vi "Set Properties.vi"(5 "Group name":string, 7 "Channel name":string, 8 "error in":errorcluster, 9 "Property values":variant[](array[variant]), 10 "Property names":string[](array[string])) -> (0 "error out":errorcluster)   [LabVIEW 2024, in "Data Logger v2.lvlib"]
doc: "Sets the properties of the TDMS file. If group and channel are no values, properties are set at the file level. If channel is empty, properties are set on the group level.\n\n_____\nCreated using DQMH Framework: Event Scripter 7.1.1.1528."
uses:
  Data Logger v2.lvlib
  Set Properties Argument--cluster.ctl
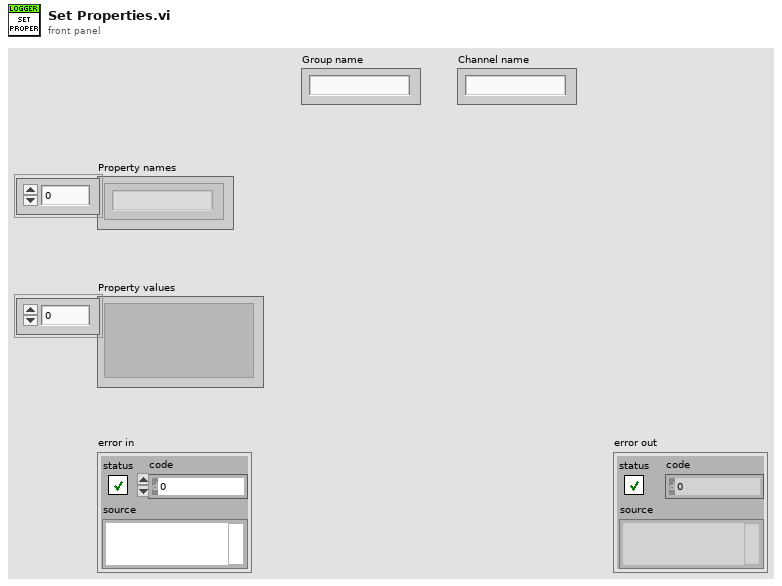
[diagram p1: front panel]
types:
  T1 = typedef "Data Logger v2.lvlib/Set Properties Argument--cluster.ctl" = cluster{"Property names":string[], "Property values":variant[], "Group name":string, "Channel name":string}
  T2 = typedef "Data Logger v2.lvlib/Request Events--cluster.ctl" = cluster{"Stop Module":refnum<user-event>, "Show Panel":refnum<user-event>, "Hide Panel":refnum<user-event>, "Get Module Execution Status":refnum<user-event>, "Show Diagram":refnum<user-event>, "Change Panel":refnum<user-event>, "Create New TDMS Log File":refnum<user-event>, "Write 2D Array to TDMS Log File":refnum<user-event>, "Close TDMS File":refnum<user-event>, "Write TDMS 2D String Array":refnum<user-event>, "Set Root Folder Path":refnum<user-event>, "Create New TDMS Log File (Relative Path)":refnum<user-event>, "Set Properties":refnum<user-event>}
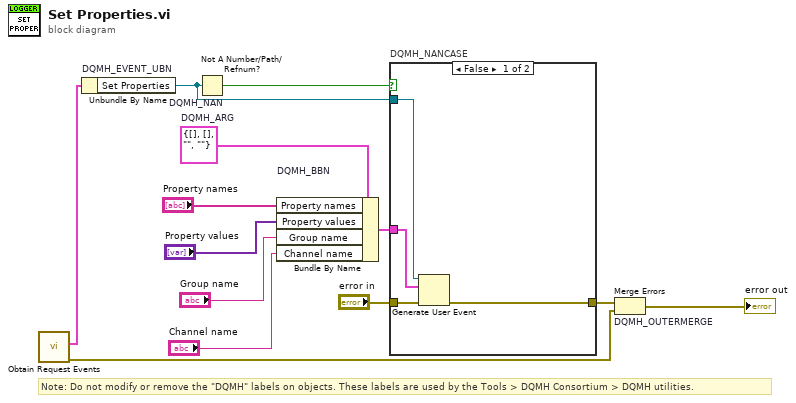
[diagram p0: block diagram]
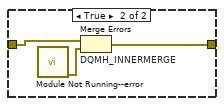
[diagram p2: hidden frame]
diagram:
  w7 = T1 {"Property names"=[], "Property values"=[], "Group name"="", "Channel name"=""}  # DQMH_ARG
  # "Note: Do not modify or remove the \"DQMH\" labels on objects. These labels are used by the Tools > DQMH Consortium > DQMH utilities."
  n1 = call "Obtain Request Events.vi"() -> ("error out"=w2:errorcluster, "Data Logger v2 Request Events"=w1:T2)  [unwired: 10 in]
  n2 = Unbundle By Name "DQMH_EVENT_UBN"(w1) -> ("Set Properties"=w9:refnum<user-event>)
  n3 = Not A Number/Path/Refnum? "DQMH_NAN"(number/path/refnum=w9) -> (NaN/Path/Refnum?=w10:bool)
  n4 = Bundle By Name "DQMH_BBN"(cluster=w7, "Property names"="Property names", "Property values"="Property values", "Group name"="Group name", "Channel name"="Channel name") -> (w11:T1)
  n5 = case "DQMH_NANCASE" shown="False" w10 {
    tunnel: "error in" -> [w17 w20]
    tunnel: [w16 w19] -> w8
    tunnel: w9 -> [w15 _]
    tunnel: w11 -> [w14 _]
    frame False {
      n6 = Generate User Event(user event=w15, event data cluster=w14, error in=w17) -> (error out=w16:errorcluster)  [unwired: 1 in, 1 out]
    }
    frame True {
      n7 = call "Module Not Running--error.vi"() -> ("error out"=w18:errorcluster)  [unwired: 11 in]
      n8 = Merge Errors "DQMH_INNERMERGE"(w20, w18) -> (w19:errorcluster)
    }
  }
  n9 = Merge Errors "DQMH_OUTERMERGE"(w8, w2) -> (→"error out":errorcluster)
